vi "NI VeriStand - Reserve Stimulus Profile Manager.vi"(8 "error in (no error)":errorcluster, 11 "StimulusProfileManager in":T1) -> (0 "error out":errorcluster, 3 "StimulusProfileManager out":T1)   [LabVIEW 2020, in "NI_VS Stimulus ExecutionAPI.lvlib"]
doc: "This VI interfaces with the legacy Stimulus Profile Editor workspace tool in NI VeriStand, and is included for compatibility only. National Instruments recommends you use the current Stimulus Profile VIs to create, observe, and control NI VeriStand stimulus profiles and real-time sequences.\n\nReserves the stimulus profile manager and prevents other clients from running stimulus profile files."
uses:
  <vilib>/NI VeriStand/Execution/Stimulus/NI_VS Stimulus ExecutionAPI.lvlib
  <vilib>/NI VeriStand/Execution/Stimulus/StimulusAPI.ctl
  NationalInstruments.VeriStand.ClientAPI
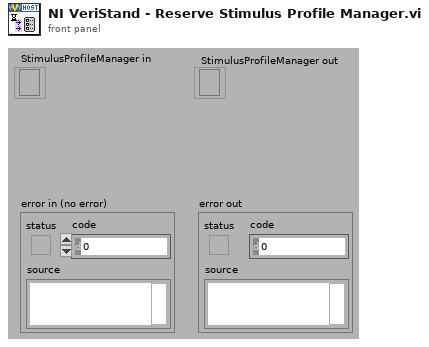
[diagram p1: front panel]
types:
  T1 = typedef "NI_VS Stimulus ExecutionAPI.lvlib/StimulusAPI.ctl" = refnum<k24>
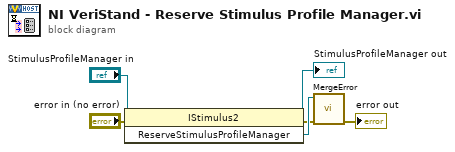
[diagram p0: block diagram]
diagram:
  n1 = invoke class="IStimulus2" method="ReserveStimulusProfileManager"(reference="StimulusProfileManager in", error in="error in (no error)") -> (reference out=→"StimulusProfileManager out":T1, error out=w2:errorcluster, "ReserveStimulusProfileManager"=w3:refnum<k24>)  [unwired: 1 in]
  n2 = call <vilib>:"MergeError.vi"("error in (no error)"=w2, "Error"=w3) -> ("error out"=→"error out":errorcluster)  [unwired: 9 out]
